vi "Generate OpenSSL Configuration File.vi"(8 "error in (no error)":errorcluster, 11 "Cert Info":T1) -> (0 "error out":errorcluster, 3 "OpenSSL Cert Config File":string)   [LabVIEW 2013, in "Certificate Generation.lvlib"]
uses:
  Certificate Generation.lvlib
  Certificate Info.ctl
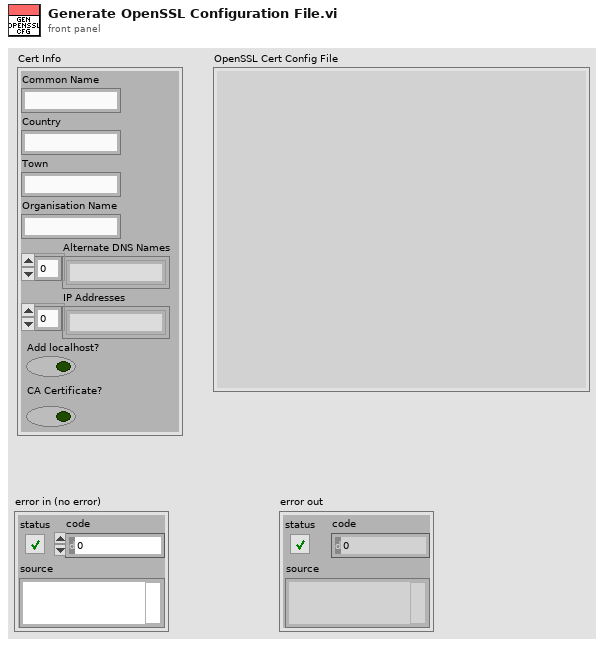
[diagram p1: front panel]
types:
  T1 = typedef "Certificate Generation.lvlib/Certificate Info.ctl" = cluster{"Common Name":string, "Country":string, "Town":string, "Organisation Name":string, "Alternate DNS Names":string[], "IP Addresses":string[], "Add localhost?":bool, "CA Certificate?":bool}
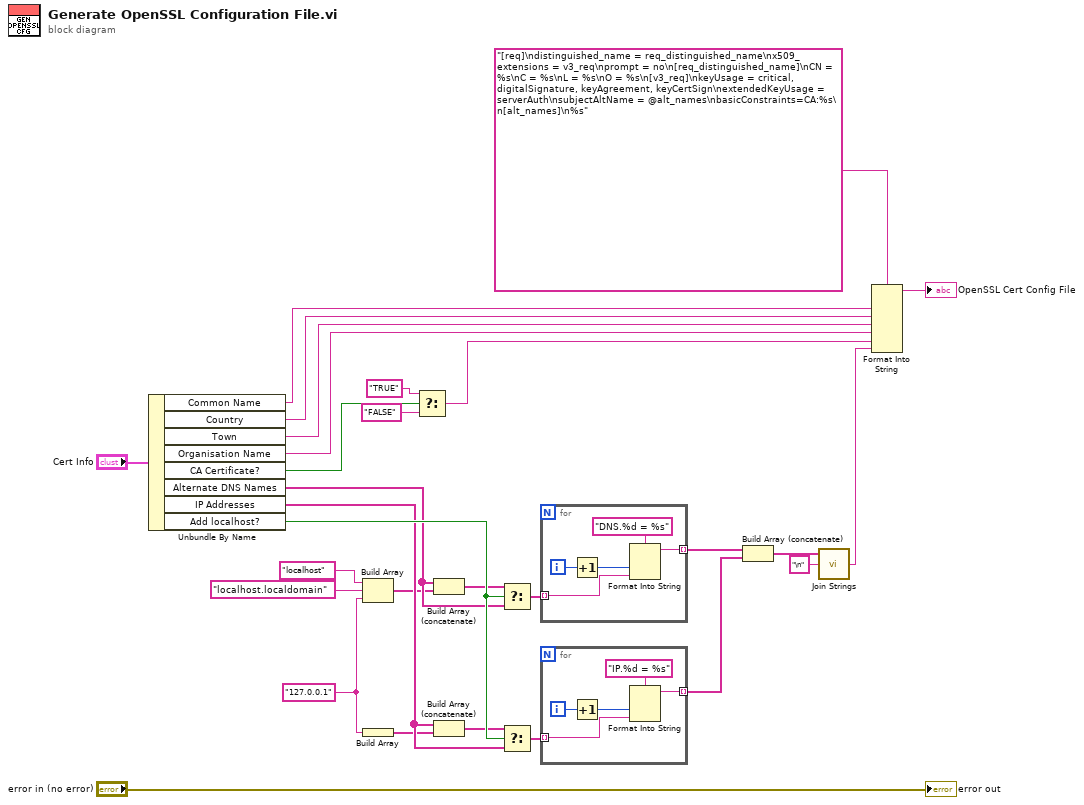
[diagram p0: block diagram]
diagram:
  w14 = "127.0.0.1"
  n1 = Unbundle By Name("Cert Info") -> ("Common Name"=w8:string, "Country"=w7:string, "Town"=w6:string, "Organisation Name"=w5:string, "CA Certificate?"=w4:bool, "Alternate DNS Names"=w26:string[], "IP Addresses"=w27:string[], "Add localhost?"=w28:bool)
  n2 = Build Array("localhost", "localhost.localdomain", w14) -> (w19:string[])
  n3 = Build Array(w14) -> (w15:string[])
  n4 = Select(t="TRUE", s=w4, f="FALSE") -> (s? t:f=w1:string)
  n5 = Build Array (concatenate)(w26, w19) -> (w18:string[])
  n6 = Build Array (concatenate)(w27, w15) -> (w16:string[])
  n7 = Select(t=w18, s=w28, f=w26) -> (s? t:f=w20:string[])
  n8 = Select(t=w16, s=w28, f=w27) -> (s? t:f=w17:string[])
  n9 = for {
    tunnel: w20 -> [w32] mode=indexing
    tunnel: [w30] -> w10 mode=indexing
    i -> [w34]
    n10 = Increment(x=w34) -> (x+1=w33:i32)
    n11 = Format Into String(format string="DNS.%d = %s", w33, w32) -> (resulting string=w30:string)  [unwired: 2 in, 1 out]
  }
  n12 = for {
    tunnel: w17 -> [w37] mode=indexing
    tunnel: [w35] -> w22 mode=indexing
    i -> [w39]
    n13 = Increment(x=w39) -> (x+1=w38:i32)
    n14 = Format Into String(format string="IP.%d = %s", w38, w37) -> (resulting string=w35:string)  [unwired: 2 in, 1 out]
  }
  n15 = Build Array (concatenate)(w10, w22) -> (w21:string[])
  n16 = call <vilib>:"Join Strings.vi"("Separator (,)"="\n", "Strings In"=w21) -> ("String"=w24:string)  [unwired: 1 in]
  n17 = Format Into String(format string="[req]\ndistinguished_name = req_distinguished_name\nx509_extensions = v3_req\nprompt = no\n[req_distinguished_name]\nCN = %s\nC = %s\nL = %s\nO = %s\n[v3_req]\nkeyUsage = critical, digitalSignature, keyAgreement, keyCertSign\nextendedKeyUsage = serverAuth\nsubjectAltName = @alt_names\nbasicConstraints=CA:%s\n[alt_names]\n%s", w8, w7, w6, w5, w1, w24) -> (resulting string=→"OpenSSL Cert Config File":string)  [unwired: 2 in, 1 out]
  "error out" <- "error in (no error)"
